vi "DIO Block Read Bank.vi"(8 "DI.DMA_ENA":T1, 9 "DATA IN":fxp<+,20,20>, 10 "DI.DMA_CNTR":u16, 11 "DMA FIFO In":refnum<k21>="DI") -> (0 "DI.DMA_IDL":bool)   [LabVIEW 2019]
uses:
  Utilities/Start Boolean.ctl
  <vilib>/rvi/DataTransferAndStorage/Container/Common/niFpgaContainerExecOnDevCompGetState.vi
  <vilib>/rvi/Emulation/niFpgaEmulationIsFPGAContextNoSignature.vi
  <vilib>/rvi/Emulation/niFpgaSctlEmulationGetInTimedLoop.vi
  <vilib>/rvi/errors/niFpgaSetErrorForExecOnDevCompSimple.vi
  <vilib>/rvi/eio/common/nirviEmuReportErrorAndStop.vi
  <vilib>/rvi/DataTransferAndStorage/Container/Common/niFpgaContainerGetUniqueNameForEmu.vi
  <vilib>/rvi/FIFO/Fifo_Resource/nirvififoEmulationSetSize.vi
  <vilib>/rvi/FIFO/Fifo_Resource/nirviFifoEmulationQueueMgr.vi
  <instcachedir>/0/nirviFifoEmulationQueueMgr_E5CAEC123FF24DC58D834DCA3CDAA9B5.lvgen/nirviFifoEmulationQueueMgr_E5CAEC123FF24DC58D834DCA3CDAA9B5_001.vi
  <vilib>/rvi/FIFO/Fifo_Resource/nirvififoEmulationDetermineInputValidOut.vi
  <vilib>/rvi/FIFO/Fifo_Resource/nirvififoEmulationCreateLock.vi
  <vilib>/rvi/Emulation/niFpgaProcessEmulError.vi
  <vilib>/rvi/FIFO/Fifo_Resource/nirvififoEmulationObtainLock.vi
  <vilib>/rvi/FIFO/Fifo_Resource/nirvififoEmulationReleaseLock.vi
  <vilib>/rvi/occurrence/nirviWaitOnOccurrenceBase.vi
  <vilib>/rvi/errors/nirviReportUnexpectedCaseInternalError.vi
  <vilib>/rvi/errors/nirviReportUnexpectedCaseInternalError (U32).vi
  <vilib>/Utility/error.llb/Clear Errors.vi
  <vilib>/rvi/interface/RandomDataEmulation/niFpgaRandomDataHandleErrors.vi
  <vilib>/rvi/DataTransferAndStorage/Container/XNode/niFpgaContainer.xnode
  <vilib>/rvi/FIFO/Fifo_Resource/niFpgaFifoEmulationRefIn.vi
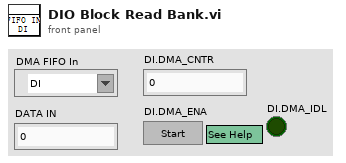
[diagram p1: front panel]
types:
  T1 = typedef "Start Boolean.ctl" = bool
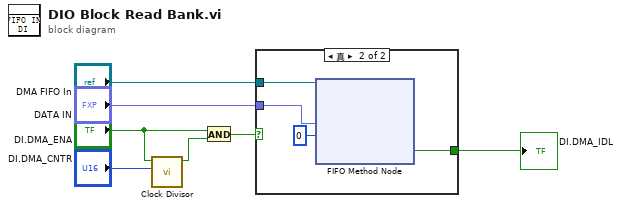
[diagram p0: block diagram]
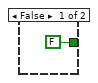
[diagram p2: hidden frame]
diagram:
  n1 = call "Clock Divisor.vi"("Count Number"="DI.DMA_CNTR", "Trigger"="DI.DMA_ENA") -> ("Finished"=w5:bool)  [unwired: 9 in]
  n2 = And(x="DI.DMA_ENA", y=w5) -> (x .and. y?=w4:T1)
  n3 = case shown="真" w4 {
    tunnel: "DMA FIFO In" -> [_ w12]
    tunnel: "DATA IN" -> [_ w11]
    tunnel: [FALSE ("Timed Out?") w9] -> w1
    frame False {
    }
    frame True {
      n4 = xnode ("FIFO Method Node")("元素"=w11, "超时"=0 ("Timeout"), "FIFO输入"=w12) -> ("超时？"=w9:bool)  [unwired: 1 out]
    }
  }
  "DI.DMA_IDL" <- w1
